vi "Read Jitter Measurement (N-Period).vi"(7 "Number of Periods (1)":i32=1, 8 "error in (no error)":errorcluster, 9 "Slope N-Period (0: Rising)":u16(ring) items=["Rising", "Falling"], 10 "Source N-Period (0: Channel 1)":u16(ring) items=["Channel 1", "Channel 2", "Channel 3", "Channel 4", "Math 1", "Math 2", "Math 3", "Math 4", "Reference Waveform 1", "Reference Waveform 2", "Reference Waveform 3", "Reference Waveform 4"], 11 "VISA resource name":refnum<visa-resource-name>) -> (0 "error out":errorcluster, 2 "N-Period":dbl, 3 "VISA resource name out":refnum<visa-resource-name>)   [LabVIEW 2023, in "Keysight-DSQx3014T.lvlib"]
doc: "Measures and returns the N-Period jitter value.\n\n<b>Note:</b>\nThis VI is specific to the 6000-X Series oscilloscopes. These features are not available on other models."
uses:
  Keysight-DSQx3014T.lvlib
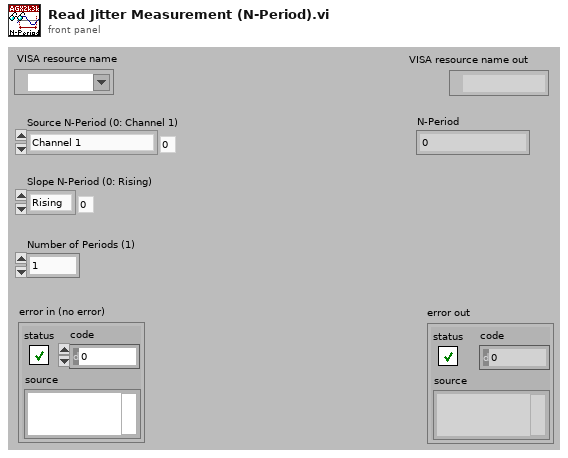
[diagram p1: front panel]
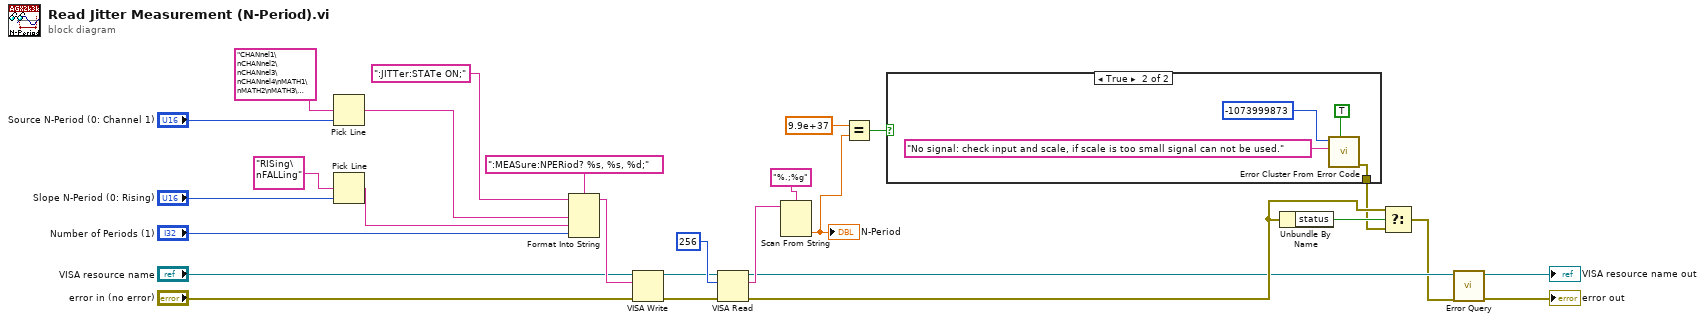
[diagram p0: block diagram]
diagram:
  n1 = Pick Line(multi-line string="CHANnel1\nCHANnel2\nCHANnel3\nCHANnel4\nMATH1\nMATH2\nMATH3\nMATH4\nWMEMory1\nWMEMory2\nWMEMory3\nWMEMory4", line index="Source N-Period (0: Channel 1)") -> (output string=w23:string)  [unwired: 1 in]
  n2 = Pick Line(multi-line string="RISing\nFALLing", line index="Slope N-Period (0: Rising)") -> (output string=w20:string)  [unwired: 1 in]
  n3 = Format Into String(format string=":MEASure:NPERiod? %s, %s, %d;", initial string=":JITTer:STATe ON;", w23, w20, "Number of Periods (1)") -> (resulting string=w19:string)  [unwired: 1 in, 1 out]
  n4 = VISA Write(VISA resource name="VISA resource name", write buffer=w19, error in (no error)="error in (no error)") -> (VISA resource name out=w5:refnum<visa-resource-name>, error out=w4:errorcluster)  [unwired: 1 out]
  n5 = VISA Read(VISA resource name=w5, byte count=u32 256, error in (no error)=w4) -> (VISA resource name out=w3:refnum<visa-resource-name>, read buffer=w14:string, error out=w8:errorcluster)  [unwired: 1 out]
  n6 = Scan From String(format string="%.;%g", input string=w14) -> (output 1=w10:dbl)  [unwired: 3 in, 3 out]
  "N-Period" <- w10
  n7 = Equal?(x=9.9e+37, y=w10) -> (x = y?=w12:bool)
  n8 = case shown="True" w12 {
    tunnel: [_ w28] -> w7
    frame False {
    }
    frame True {
      n9 = call <vilib>:"Error Cluster From Error Code.vi"("show call chain? (False)"=TRUE, "error message (\"\")"="No signal: check input and scale, if scale is too small signal can not be used." ("error message (\"\")"), "error code (0)"=-1073999873) -> ("error out"=w28:errorcluster)  [unwired: 6 in]
    }
  }
  n10 = Unbundle By Name(w8) -> ("status"=w9:bool)
  n11 = Select(t=w8, s=w9, f=w7) -> (s? t:f=w2:errorcluster)
  n12 = call "Error Query.vi"("error in (no error)"=w2, "VISA resource name"=w3) -> ("error out"=→"error out":errorcluster, "VISA resource name out"=→"VISA resource name out":refnum<visa-resource-name>)  [unwired: 6 in, 2 out]
